vi "AB_860_900_Project_Source_RESTfulVI.vi"(7 "action":T3, 8 "error in (no error)":errorcluster, 9 "index in":i32, 10 "dataSource in":T1={"RESTful VI configuration"={"Service VI Type"=enum."Web Method", "Load VI at statup"=TRUE, "Keep VI in memory"=TRUE, "Output type"=enum."Terminal", "Output format"=enum."XML", "Use headers"=TRUE, "Buffered"=TRUE}}, 11 "buildObject":T2) -> (0 "error out":errorcluster, 1 "index out":i32, 2 "dataSource out":T1={"RESTful VI configuration"={"Service VI Type"=enum."Web Method", "Load VI at statup"=TRUE, "Keep VI in memory"=TRUE, "Output type"=enum."Terminal", "Output format"=enum."XML", "Use headers"=TRUE, "Buffered"=TRUE}}, 3 "buildObject out":T2)   [LabVIEW 2020]
doc: "Reads and writes the data to the object property bag."
uses:
  <resource>/Framework/Providers/API/ItemRef.ctl
  <vilib>/AppBuilder/RW_Project/AB_RW_Project_PropBag_Action.ctl
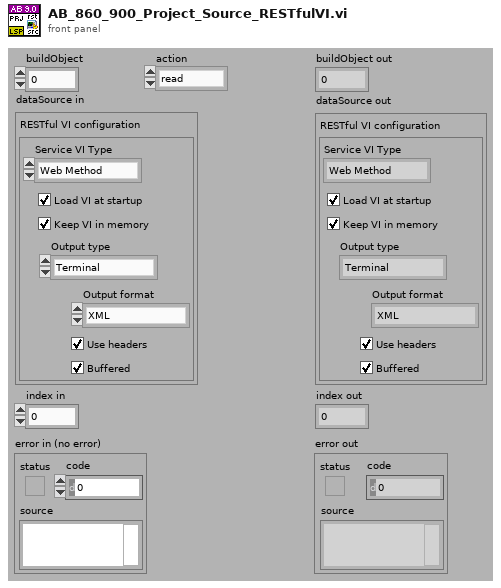
[diagram p1: front panel]
types:
  T1 = cluster{"RESTful VI configuration":cluster{"Service VI Type":enum32{"Web Method", "Auxiliary"}, "Load VI at statup":bool, "Keep VI in memory":bool, "Output type":enum32{"Terminal", "Stream"}, "Output format":enum32{"XML", "Text", "HTML", "JSON"}, "Use headers":bool, "Buffered":bool}}
  T2 = typedef "ItemRef.ctl" = u64
  T3 = typedef "AB_RW_Project_PropBag_Action.ctl" = enum16{"read", "write", "clear", "readPrevious", "writePrevious", "clearPrevious"}
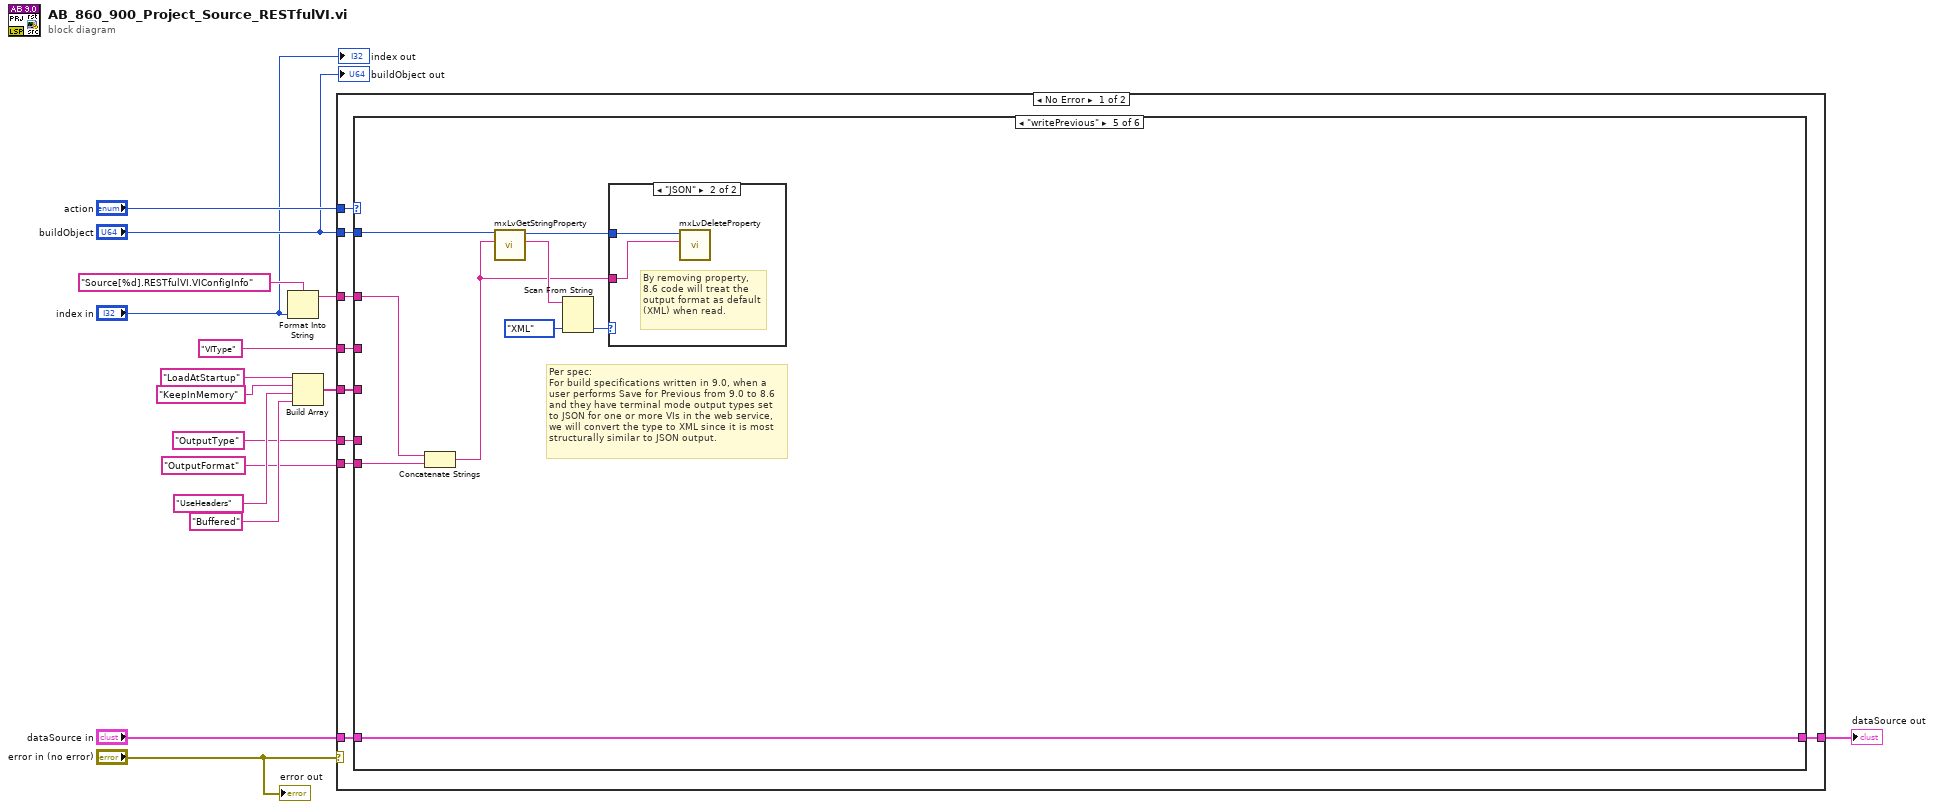
[diagram p0: block diagram]
diagram:
  n1 = Format Into String(format string="Source[%d].RESTfulVI.VIConfigInfo", "index in") -> (resulting string=w14:string)  [unwired: 2 in, 1 out]
  n2 = Build Array("LoadAtStartup", "KeepInMemory", "UseHeaders", "Buffered") -> (w2:string[])
  n3 = case shown="No Error" "error in (no error)" {
    tunnel: "action" -> [w25 _]
    tunnel: "dataSource in" -> [w24 w42]
    tunnel: w14 -> [w23 _]
    tunnel: "buildObject" -> [w22 _]
    tunnel: [w21 w42] -> w9
    tunnel: "VIType" -> [w20 _]
    tunnel: "OutputType" -> [w19 _]
    tunnel: "OutputFormat" -> [w18 _]
    tunnel: w2 -> [w17 _]
    frame No Error {
      n4 = case shown="\"writePrevious\"" w25 {
        tunnel: w22 -> [_ _ _ _ w33 _]
        tunnel: w24 -> [w26 w27 w28 w29 w38 w41]
        tunnel: w23 -> [_ _ _ _ w36 _]
        tunnel: [w26 w27 w28 w29 w38 w41] -> w21
        tunnel: w20 -> [_ _ _ _ _ _]
        tunnel: w19 -> [_ _ _ _ _ _]
        tunnel: w18 -> [_ _ _ _ w35 _]
        tunnel: w17 -> [_ _ _ _ _ _]
        frame "read" {
        }
        frame "write" {
        }
        frame "clear" {
        }
        frame "readPrevious" {
        }
        frame "writePrevious" {
          # "Per spec:\nFor build specifications written in 9.0, when a user performs Save for Previous from 9.0 to 8.6 and they have terminal mode output types set to JSON for one or more VIs in the web service, we will convert the type to XML since it is most structurally similar to JSON output."
          n5 = Concatenate Strings(w36, w35) -> (w30:string)
          n6 = call <resource>:"mxLvGetStringProperty.vi"("Tag"=w30, "Item"=w33) -> ("Value"=w34:string, "Item"=w31:T2)  [unwired: 1 in, 7 out]
          n7 = Scan From String(input string=w34, default 1=enum32{"XML", "Text", "HTML", "JSON"}."XML" ("Output format")) -> (output 1=w32:enum32{"XML", "Text", "HTML", "JSON"})  [unwired: 3 in, 3 out]
          n8 = case shown="\"JSON\"" w32 {
            tunnel: w31 -> [_ w40]
            tunnel: w30 -> [_ w39]
            frame Default {
            }
            frame "JSON" {
              # "By removing property, 8.6 code will treat the output format as default (XML) when read."
              n9 = call <resource>:"mxLvDeleteProperty.vi"("Tag"=w39, "Item"=w40) -> ()  [unwired: 2 in, 8 out]
            }
          }
        }
        frame "clearPrevious" {
        }
      }
    }
    frame Error {
    }
  }
  "dataSource out" <- w9
  "error out" <- "error in (no error)"
  "buildObject out" <- "buildObject"
  "index out" <- "index in"
